vi "Blend.vi"(7 "Source Name in":string, 8 "error in (no error)":errorcluster, 9 "Source Enqueuer":refnum<class "Message Enqueuer.lvclass">, 10 "Sample to Blend in":refnum<class "Sample.lvclass">, 11 "Storage Line in":refnum<class "Storage Line.lvclass">) -> (0 "error out":errorcluster, 2 "Source Name":string, 3 "Storage Line out":refnum<class "Storage Line.lvclass">)   [LabVIEW 2015, in "cRIO-Carbondioxide.lvlib" / "CO2-Actor.lvlib" / "Storage Line.lvclass"]
uses:
  Storage Line.lvclass
  subs/Sample/Sample.lvclass
  <vilib>/ActorFramework/Message Enqueuer/Message Enqueuer.lvclass
  Storage Line.lvclass/Storage Line.ctl
  Read Container.vi
  CO2 Actor/CO2 Actor.lvclass
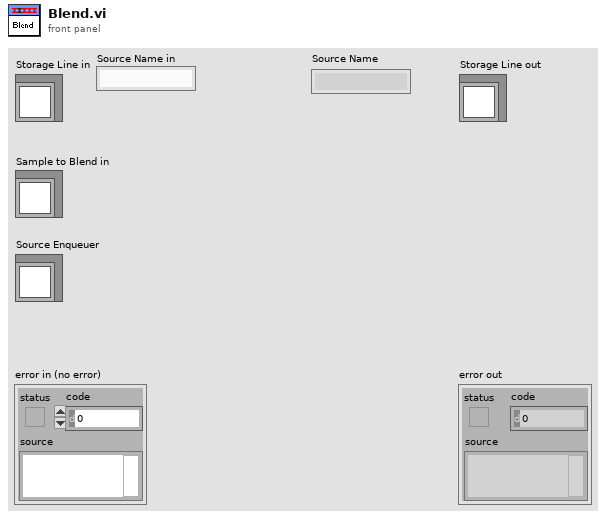
[diagram p1: front panel]
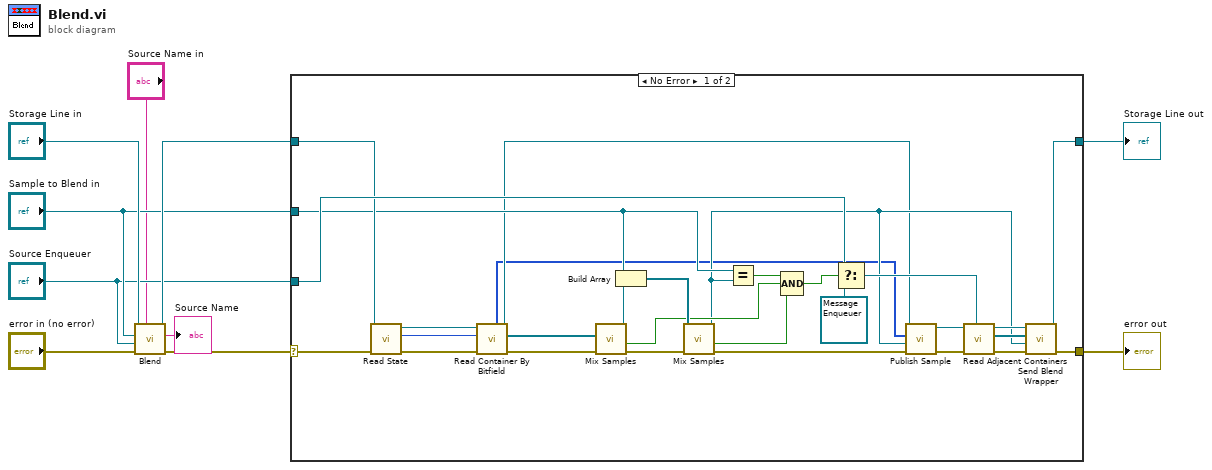
[diagram p0: block diagram]
diagram:
  n1 = call-parent "Blend.vi"("Source Name in"="Source Name in", "error in (no error)"="error in (no error)", "Source Enqueuer"="Source Enqueuer", "Sample to Blend in"="Sample to Blend in", "CO2 Actor in"="Storage Line in") -> ("error out"=w8:errorcluster, "Source Name"=→"Source Name":string, "CO2 Actor out"=w5:refnum<class "Storage Line.lvclass">)  [unwired: 4 in]
  n2 = case shown="No Error" w8 {
    selector: w8 -> [w39 w41]
    tunnel: [w32 w41] -> w7
    tunnel: [w30 w40] -> w6
    tunnel: w5 -> [w33 w40]
    tunnel: "Sample to Blend in" -> [w22 _]
    tunnel: "Source Enqueuer" -> [w38 _]
    frame No Error {
      n3 = call "Read State.vi"("error in (no error)"=w39, "Storage Line in"=w33) -> ("error out"=w15:errorcluster, "State"=w16:u16, "Storage Line out"=w17:refnum<class "Storage Line.lvclass">)  [unwired: 5 in, 2 out]
      n4 = call "Read Container By Bitfield.vi"("error in (no error)"=w15, "Bitfield"=w16, "Storage Line in"=w17) -> ("error out"=w14:errorcluster, "Samples"=w13:refnum<class "Sample.lvclass">[], "Storage Line out"=w12:refnum<class "Storage Line.lvclass">, "Indice"=w11:i32[])  [unwired: 4 in, 1 out]
      n5 = call "Mix Samples.vi"("error in (no error)"=w14, "Samples In"=w13) -> ("error out"=w27:errorcluster, "is clean?"=w23:bool, "Sample out"=w26:refnum<class "Sample.lvclass">)  [unwired: 6 in, 1 out]
      n6 = Build Array(w22, w26) -> (w25:refnum<class "Sample.lvclass">[])
      n7 = call "Mix Samples.vi"("error in (no error)"=w27, "Samples In"=w25) -> ("error out"=w21:errorcluster, "is clean?"=w24:bool, "Sample out"=w20:refnum<class "Sample.lvclass">)  [unwired: 6 in, 1 out]
      n8 = Equal?(x=w22, y=w20) -> (x = y?=w29:bool)
      n9 = Compound Arithmetic op=AND(w29, w23, w24) -> (w28:bool)
      n10 = Select(t=w38, s=w28, f=refnum<class "Message Enqueuer.lvclass"> refnum) -> (s? t:f=w37:refnum<class "Message Enqueuer.lvclass">)
      n11 = call "Publish Sample.vi"("error in (no error)"=w21, "Sample"=w20, "Indice"=w11, "Storage Line in"=w12) -> ("error out"=w18:errorcluster, "Storage Line out"=w19:refnum<class "Storage Line.lvclass">)  [unwired: 6 in]
      n12 = call "Read Adjacent Containers.vi"("Exclude Source"=w37, "error in (no error)"=w18, "Storage Line in"=w19) -> ("error out"=w35:errorcluster, "Adjacent Containers"=w34:refnum<class "Message Enqueuer.lvclass">[], "Storage Line out"=w31:refnum<class "Storage Line.lvclass">)  [unwired: 6 in]
      n13 = call-dynamic "Send Blend Wrapper.vi"("error in (no error)"=w35, "Sample to Blend"=w20, "Send to"=w34, "CO2 Actor in"=w31) -> ("error out"=w32:errorcluster, "CO2 Actor out"=w30:refnum<class "Storage Line.lvclass">)  [unwired: 6 in]
    }
    frame Error {
    }
  }
  "error out" <- w7
  "Storage Line out" <- w6
